vi "MessageProbe.vi"(1 "Message":refnum<class "MSG.lvclass">) -> (0 "Boolean":bool)   [LabVIEW 2011, in "Messenging.lvlib"]
uses:
  Messenging.lvlib
  Interprocess Messenger/TextVarientMessage/MSG.lvclass
  Interprocess Messenger/Send/Send.lvclass
panel:
  out "Table":string[][](table)
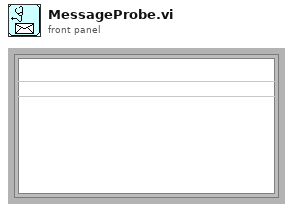
[diagram p1: front panel]
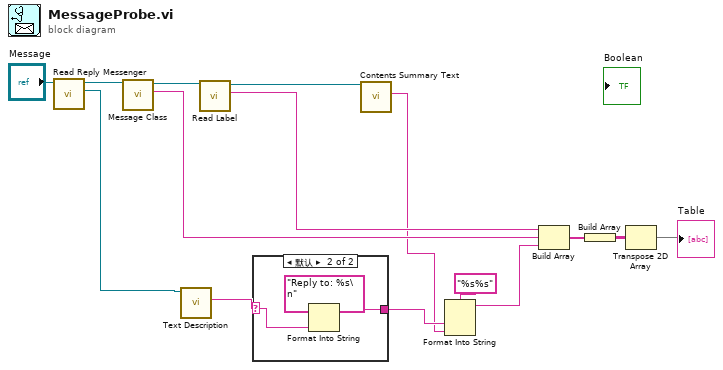
[diagram p0: block diagram]
diagram:
  n1 = call-dynamic "Read Reply Messenger.vi"("Messege"="Message") -> ("Reply to..."=w2:refnum<class "Send.lvclass">, "Message"=w7:refnum<class "MSG.lvclass">)  [unwired: 1 in, 8 out]
  n2 = call-dynamic "Message Class.vi"("Message"=w7) -> ("Message Class"=w12:string, "Message"=w15:refnum<class "MSG.lvclass">)  [unwired: 1 in, 8 out]
  n3 = call-dynamic "Text Description.vi"("Send in"=w2) -> ("Description"=w1:string)  [unwired: 10 out]
  n4 = call-dynamic "Read Label.vi"("Message"=w15) -> ("Label"=w13:string, "Message"=w14:refnum<class "MSG.lvclass">)  [unwired: 1 in, 8 out]
  n5 = case shown="默认" w1 {
    selector: w1 -> [w16 w17]
    tunnel: [w16 w19] -> w5
    frame "" {
    }
    frame Default {
      n6 = Format Into String(format string="Reply to: %s\n", w17) -> (resulting string=w19:string)  [unwired: 2 in, 1 out]
    }
  }
  n7 = call-dynamic "Contents Summary Text.vi"("Message"=w14) -> ("Contents Summary Text"=w4:string)  [unwired: 10 out]
  n8 = Format Into String(format string="%s%s", w5, w4) -> (resulting string=w3:string)  [unwired: 2 in, 1 out]
  n9 = Build Array(w13, w12, w3) -> (w11:string[])
  n10 = Build Array(w11) -> (w10:string[][])
  n11 = Transpose 2D Array(2D array=w10) -> (transposed array=→"Table":string[][])
